vi "Config Mgr DVR.vi"(4 "Error In":errorcluster) -> (0 "Error Out":errorcluster, 3 "DVR":refnum<data-value>)   [LabVIEW 2014, in "Config Data.lvlib" / "Config Data.lvclass"]
uses:
  Config Data.lvclass
  Config Mgr Data.ctl
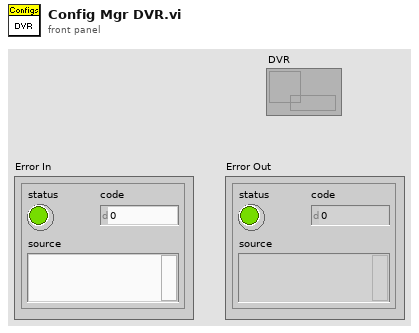
[diagram p1: front panel]
types:
  T1 = typedef "Config Data.lvlib/Config Data.lvclass/Config Mgr Data.ctl" = cluster{"User ID":string, "Password":string}
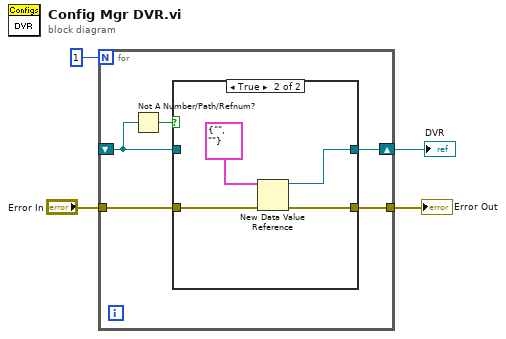
[diagram p0: block diagram]
diagram:
  n1 = for {
    N: 1 -> [_]
    shift-right: [w9] -> w1
    shift-left: _ -> [w8]
    tunnel: [w6] -> w3
    tunnel: "Error In" -> [w5]
    n2 = Not A Number/Path/Refnum?(number/path/refnum=w8) -> (NaN/Path/Refnum?=w7:bool)
    n3 = case shown="True" w7 {
      tunnel: [w11 w12] -> w9
      tunnel: w8 -> [w11 _]
      tunnel: [w10 w13] -> w6
      tunnel: w5 -> [w10 w14]
      frame False {
      }
      frame True {
        n4 = New Data Value Reference(data value=T1 {"User ID"="", "Password"=""} ("Config Manager Data"), error in=w14) -> (data value reference=w12:refnum<data-value>, error out=w13:errorcluster)
      }
    }
  }
  "Error Out" <- w3
  "DVR" <- w1
